vi "TEST - Delete Elements from 2D Array.vi"(8 "error in (no error)":errorcluster) -> (0 "error out":errorcluster, 2 "Pass?":bool=TRUE)   [LabVIEW 2009]
doc: "This VI template can be used for the functional testing of VIs; this implementation includes handling for the testing of polymorphic VIs, and the polymorphic elements should be removed if not needed.\n\nCoded by Douglas A. Femec, January 24, 2006.\n\nCopyright (c) 2005-2006 MKS Instruments, Inc.\nAll rights reserved."
uses:
  TEST - Delete Elements from 2D Array - Inputs.ctl
  Polymorphizer+ Data Type.ctl
  TEST - Delete Elements from 2D Array - Outputs.ctl
  source/library/Delete Elements from Array/Delete Elements from 2D Array (EXT).vi
  source/library/Delete Elements from Array/Delete Elements from 2D Array (I64).vi
  source/library/Delete Elements from Array/Delete Elements from 2D Array (U64).vi
  source/library/Delete Elements from Array/Delete Elements from 2D Array (DBL).vi
  source/library/Delete Elements from Array/Delete Elements from 2D Array (SGL).vi
  source/library/Delete Elements from Array/Delete Elements from 2D Array (I32).vi
  source/library/Delete Elements from Array/Delete Elements from 2D Array (I16).vi
  source/library/Delete Elements from Array/Delete Elements from 2D Array (I8).vi
  source/library/Delete Elements from Array/Delete Elements from 2D Array (LVObject).vi
  source/library/Delete Elements from Array/Delete Elements from 2D Array (U32).vi
  source/library/Delete Elements from Array/Delete Elements from 2D Array (U16).vi
  source/library/Delete Elements from Array/Delete Elements from 2D Array (U8).vi
  source/library/Delete Elements from Array/Delete Elements from 2D Array (CXT).vi
  source/library/Delete Elements from Array/Delete Elements from 2D Array (CDB).vi
  source/library/Delete Elements from Array/Delete Elements from 2D Array (CSG).vi
  source/library/Delete Elements from Array/Delete Elements from 2D Array (Boolean).vi
  source/library/Delete Elements from Array/Delete Elements from 2D Array (String).vi
  source/library/Delete Elements from Array/Delete Elements from 2D Array (Path).vi
  source/library/Delete Elements from Array/Delete Elements from 2D Array (Variant).vi
  TestClass/TestClass.lvclass
panel:
  out "Generated Outputs":T1[][](array[typedef])=[[{"Description"="expect empty array", "array w/ subset deleted"=[], "deleted elements"=[]}, {"Description"="expect empty array", "array w/ subset deleted"=[], "deleted elements"=[]}, {"Description"="expect empty array", "array w/ subset deleted"=[], "deleted elements"=[]}, {"Description"="expect empty array", "array w/ subset deleted"=[], "deleted elements"=[]}, {"Description"="expect empty array", "array w/ subset deleted"=[], "deleted elements"=[]}, {"Description"="expect empty array", "array w/ subset deleted"=[], "deleted elements"=[]}, {"Description"="expect empty array", "array w/ subset deleted"=[], "deleted elements"=[]}, {"Description"="expect empty array", "array w/ subset deleted"=[], "deleted elements"=[]}, {"Description"="expect empty array", "array w/ subset deleted"=[], "deleted elements"=[]}, {"Description"="expect empty array", "array w/ subset deleted"=[], "deleted elements"=[]}, {"Description"="expect empty array", "array w/ subset deleted"=[], "deleted elements"=[]}, {"Description"="expect empty array", "array w/ subset deleted"=[], "deleted elements"=[]}, {"Description"="expect empty array", "array w/ subset deleted"=[], "deleted elements"=[]}, {"Description"="expect empty array", "array w/ subset deleted"=[], "deleted elements"=[]}, {"Description"="expect empty array", "array w/ subset deleted"=[], "deleted elements"=[]}, {"Description"="expect empty array", "array w/ subset deleted"=[], "deleted elements"=[]}], [{"Description"="Some rows deleted", "array w/ subset deleted"=[[3.0, 4.0], [7.0, 8.0]], "deleted elements"=[[5.0, 6.0], [1.0, 2.0]]}, {"Description"="Some rows deleted", "array w/ subset deleted"=[[3.0, 4.0], [7.0, 8.0]], "deleted elements"=[[5.0, 6.0], [1.0, 2.0]]}, {"Description"="Some rows deleted", "array w/ subset deleted"=[[3.0, 4.0], [7.0, 8.0]], "deleted elements"=[[5.0, 6.0], [1.0, 2.0]]}, {"Description"="Some rows deleted", "array w/ subset deleted"=[[3.0, 4.0], [7.0, 8.0]], "deleted elements"=[[5.0, 6.0], [1.0, 2.0]]}, {"Description"="Some rows deleted", "array w/ subset deleted"=[[3.0, 4.0], [7.0, 8.0]], "deleted elements"=[[5.0, 6.0], [1.0, 2.0]]}, {"Description"="Some rows deleted", "array w/ subset deleted"=[[3.0, 4.0], [7.0, 8.0]], "deleted elements"=[[5.0, 6.0], [1.0, 2.0]]}, {"Description"="Some rows deleted", "array w/ subset deleted"=[[3.0, 4.0], [7.0, 8.0]], "deleted elements"=[[5.0, 6.0], [1.0, 2.0]]}, {"Description"="Some rows deleted", "array w/ subset deleted"=[[3.0, 4.0], [7.0, 8.0]], "deleted elements"=[[5.0, 6.0], [1.0, 2.0]]}, {"Description"="Some rows deleted", "array w/ subset deleted"=[[3.0, 4.0], [7.0, 8.0]], "deleted elements"=[[5.0, 6.0], [1.0, 2.0]]}, {"Description"="Some rows deleted", "array w/ subset deleted"=[[3.0, 4.0], [7.0, 8.0]], "deleted elements"=[[5.0, 6.0], [1.0, 2.0]]}, {"Description"="Some rows deleted", "array w/ subset deleted"=[[3.0, 4.0], [7.0, 8.0]], "deleted elements"=[[5.0, 6.0], [1.0, 2.0]]}, {"Description"="Some rows deleted", "array w/ subset deleted"=[[3.0, 4.0], [7.0, 8.0]], "deleted elements"=[[5.0, 6.0], [1.0, 2.0]]}, {"Description"="Some rows deleted", "array w/ subset deleted"=[[3.0, 4.0], [7.0, 8.0]], "deleted elements"=[[5.0, 6.0], [1.0, 2.0]]}, {"Description"="Some rows deleted", "array w/ subset deleted"=[[3.0, 4.0], [7.0, 8.0]], "deleted elements"=[[5.0, 6.0], [1.0, 2.0]]}, {"Description"="Some rows deleted", "array w/ subset deleted"=[[3.0, 4.0], [7.0, 8.0]], "deleted elements"=[[5.0, 6.0], [1.0, 2.0]]}, {"Description"="", "array w/ subset deleted"=[], "deleted elements"=[]}], [{"Description"="", "array w/ subset deleted"=[], "deleted elements"=[]}, {"Description"="", "array w/ subset deleted"=[], "deleted elements"=[]}, {"Description"="", "array w/ subset deleted"=[], "deleted elements"=[]}, {"Description"="", "array w/ subset deleted"=[], "deleted elements"=[]}, {"Description"="", "array w/ subset deleted"=[], "deleted elements"=[]}, {"Description"="", "array w/ subset deleted"=[], "deleted elements"=[]}, {"Description"="", "array w/ subset deleted"=[], "deleted elements"=[]}, {"Description"="", "array w/ subset deleted"=[], "deleted elements"=[]}, {"Description"="", "array w/ subset deleted"=[], "deleted elements"=[]}, {"Description"="", "array w/ subset deleted"=[], "deleted elements"=[]}, {"Description"="", "array w/ subset deleted"=[], "deleted elements"=[]}, {"Description"="", "array w/ subset deleted"=[], "deleted elements"=[]}, {"Description"="", "array w/ subset deleted"=[], "deleted elements"=[]}, {"Description"="", "array w/ subset deleted"=[], "deleted elements"=[]}, {"Description"="", "array w/ subset deleted"=[], "deleted elements"=[]}, {"Description"="", "array w/ subset deleted"=[], "deleted elements"=[]}], [{"Description"="", "array w/ subset deleted"=[], "deleted elements"=[]}, {"Description"="", "array w/ subset deleted"=[], "deleted elements"=[]}, {"Description"="", "array w/ subset deleted"=[], "deleted elements"=[]}, {"Description"="", "array w/ subset deleted"=[], "deleted elements"=[]}, {"Description"="", "array w/ subset deleted"=[], "deleted elements"=[]}, {"Description"="", "array w/ subset deleted"=[], "deleted elements"=[]}, {"Description"="", "array w/ subset deleted"=[], "deleted elements"=[]}, {"Description"="", "array w/ subset deleted"=[], "deleted elements"=[]}, {"Description"="", "array w/ subset deleted"=[], "deleted elements"=[]}, {"Description"="", "array w/ subset deleted"=[], "deleted elements"=[]}, {"Description"="", "array w/ subset deleted"=[], "deleted elements"=[]}, {"Description"="", "array w/ subset deleted"=[], "deleted elements"=[]}, {"Description"="", "array w/ subset deleted"=[], "deleted elements"=[]}, {"Description"="", "array w/ subset deleted"=[], "deleted elements"=[]}, {"Description"="", "array w/ subset deleted"=[], "deleted elements"=[]}, {"Description"="", "array w/ subset deleted"=[], "deleted elements"=[]}]] {"deleted elements" format="%.2f"; "array w/ subset deleted" format="%.2f"}
  in  "Expected Outputs":T1[](array[typedef])=[{"Description"="expect empty array", "array w/ subset deleted"=[], "deleted elements"=[]}, {"Description"="Some rows deleted", "array w/ subset deleted"=[[3.0, 4.0], [7.0, 8.0]], "deleted elements"=[[5.0, 6.0], [1.0, 2.0]]}, {"Description"="", "array w/ subset deleted"=[], "deleted elements"=[]}, {"Description"="", "array w/ subset deleted"=[], "deleted elements"=[]}] {"deleted elements" format="%.2f"; "array w/ subset deleted" format="%.2f"}
  in  "Inputs":T2[](array[typedef])=[{"Description"="Empty array", "Data Types to Test"=[enum."EXT", enum."DBL", enum."SGL", enum."I32", enum."I16", enum."I8", enum."U32", enum."U16", enum."U8", enum."CXT", enum."CDB", enum."CSG", enum."Boolean", enum."String", enum."Path", enum."Variant", enum."I64", enum."U64", enum."LabVIEW Object"], "Array"=[], "Indices"=[], "delete (rows or columns)"=enum."rows"}, {"Description"="Delete some rows", "Data Types to Test"=[enum."EXT", enum."DBL", enum."SGL", enum."I32", enum."I16", enum."I8", enum."U32", enum."U16", enum."U8", enum."CXT", enum."CDB", enum."CSG", enum."String", enum."Path", enum."Variant", enum."I64", enum."U64", enum."LabVIEW Object"], "Array"=[[1.0, 2.0], [3.0, 4.0], [5.0, 6.0], [7.0, 8.0]], "Indices"=[2, 0], "delete (rows or columns)"=enum."rows"}, {"Description"="", "Data Types to Test"=[enum."EXT", enum."DBL", enum."SGL", enum."I32", enum."I16", enum."I8", enum."U32", enum."U16", enum."U8", enum."CXT", enum."CDB", enum."CSG", enum."Boolean", enum."String", enum."Path", enum."Variant", enum."I64", enum."U64", enum."LabVIEW Object"], "Array"=[], "Indices"=[], "delete (rows or columns)"=enum."rows"}, {"Description"="", "Data Types to Test"=[enum."EXT", enum."DBL", enum."SGL", enum."I32", enum."I16", enum."I8", enum."U32", enum."U16", enum."U8", enum."CXT", enum."CDB", enum."CSG", enum."Boolean", enum."String", enum."Path", enum."Variant", enum."I64", enum."U64", enum."LabVIEW Object"], "Array"=[], "Indices"=[], "delete (rows or columns)"=enum."rows"}] {"Array" format="%.2f"}
  # "Copyright (c) 2005-2006 MKS Instruments, Inc.\nAll rights reserved."
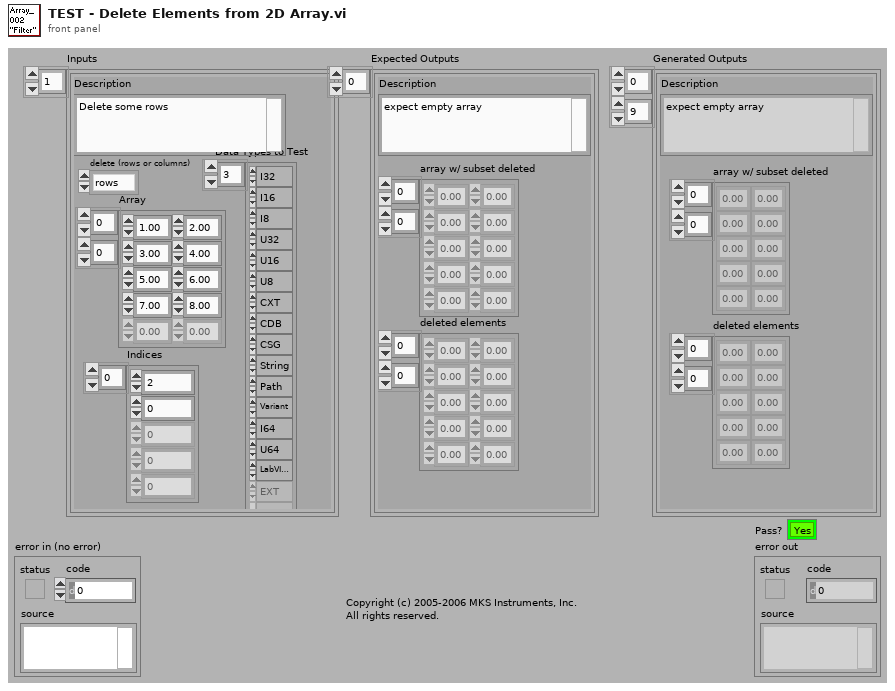
[diagram p1: front panel]
types:
  T1 = typedef "TEST - Delete Elements from 2D Array - Outputs.ctl" = cluster{"Description":string, "array w/ subset deleted":sgl[][], "deleted elements":sgl[][]}
  T2 = typedef "TEST - Delete Elements from 2D Array - Inputs.ctl" = cluster{"Description":string, "Data Types to Test":T3[], "Array":sgl[][], "Indices":i32[], "delete (rows or columns)":enum16{"rows", "columns"}}
  T3 = typedef "Polymorphizer+ Data Type.ctl" = enum16{"EXT", "DBL", "SGL", "I32", "I16", "I8", "U32", "U16", "U8", "CXT", "CDB", "CSG", "Boolean", "String", "Path", "Variant", "CTL-REF", "GEN-REF", "GObj-REF", "VI-REF", "ENUM", "ERR", "FILE-REF", "MENU-REF", "MENU-RING", "PICT-RING", "TXT&PICT-RING", "TXT-RING", "I64", "U64", "LabVIEW Object"}
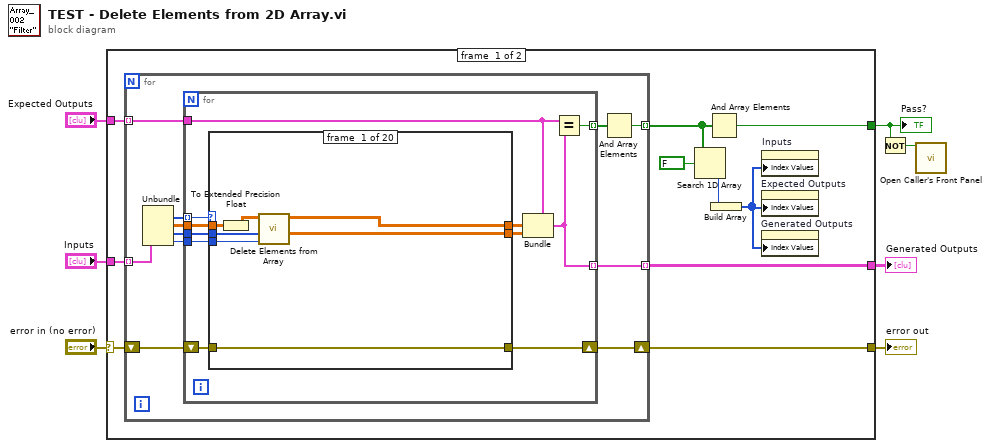
[diagram p0: block diagram]
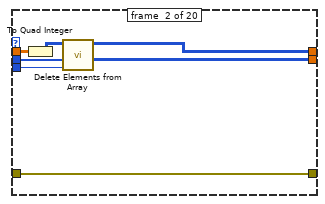
[diagram p2: hidden frame]
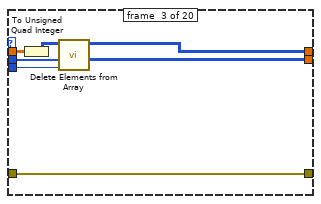
[diagram p3: hidden frame]
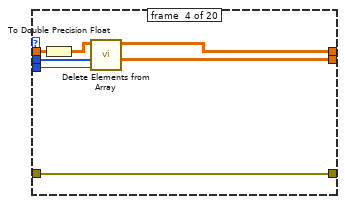
[diagram p4: hidden frame]
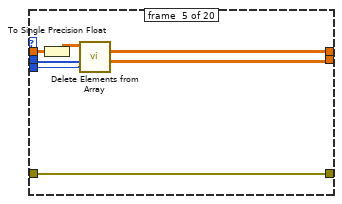
[diagram p5: hidden frame]
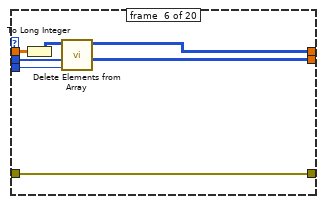
[diagram p6: hidden frame]
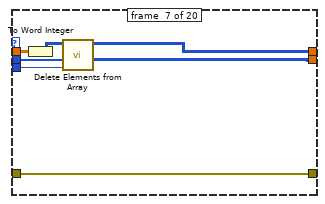
[diagram p7: hidden frame]
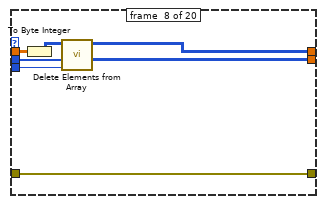
[diagram p8: hidden frame]
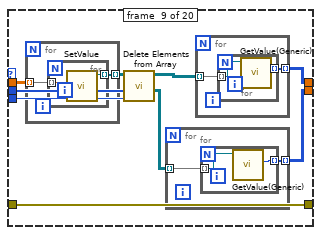
[diagram p9: hidden frame]
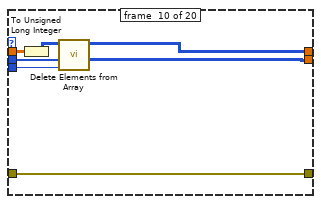
[diagram p10: hidden frame]
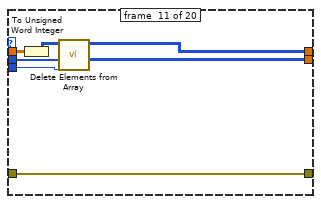
[diagram p11: hidden frame]
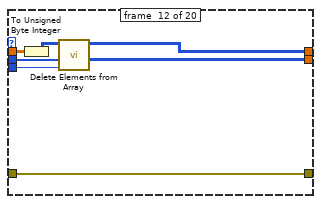
[diagram p12: hidden frame]
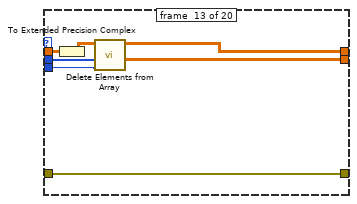
[diagram p13: hidden frame]
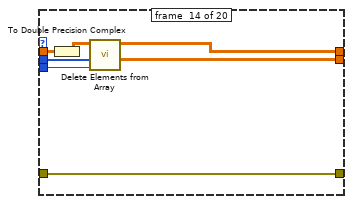
[diagram p14: hidden frame]
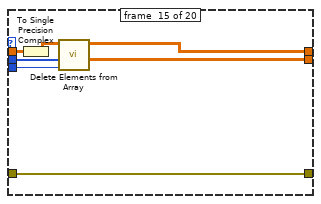
[diagram p15: hidden frame]
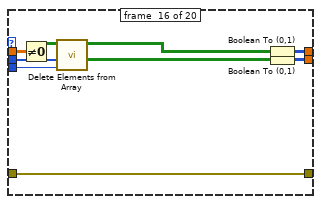
[diagram p16: hidden frame]
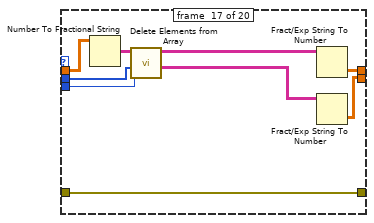
[diagram p17: hidden frame]
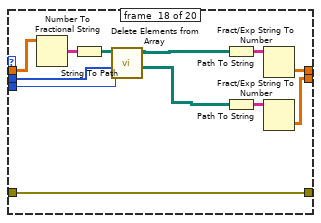
[diagram p18: hidden frame]
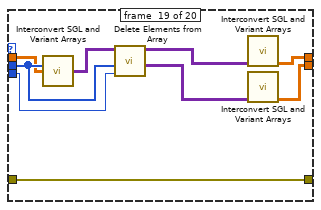
[diagram p19: hidden frame]
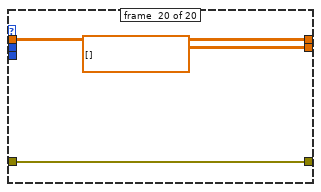
[diagram p20: hidden frame]
diagram:
  n1 = case shown="No Error" "error in (no error)" {
    selector: "error in (no error)" -> [w16 w201]
    tunnel: [w17 w201] -> w6
    tunnel: "Expected Outputs" -> [w14 _]
    tunnel: "Inputs" -> [w15 _]
    tunnel: [w13 _] -> w3
    tunnel: [w12 _] -> w2
    frame #0 {
      n2 = for {
        shift-right: [w23] -> w17
        shift-left: w16 -> [w24]
        tunnel: w15 -> [w25] mode=indexing
        tunnel: w14 -> [w28] mode=indexing
        tunnel: [w27] -> w13 mode=indexing
        tunnel: [w22] -> w11 mode=indexing
        n3 = Unbundle(w25) -> ("Data Types to Test"=w21:T3[], "Array"=w19:sgl[][], "Indices"=w20:i32[], "delete (rows or columns)"=w18:enum16{"rows", "columns"})  [unwired: 1 out]
        n4 = for {
          tunnel: w28 -> [w39]
          tunnel: [w37] -> w27 mode=indexing
          tunnel: [w38] -> w26 mode=indexing
          shift-right: [w32] -> w23
          shift-left: w24 -> [w33]
          tunnel: w21 -> [w34] mode=indexing
          tunnel: w19 -> [w36]
          tunnel: w20 -> [w35]
          tunnel: w18 -> [w29]
          n5 = case shown="\"LabVIEW Object\"" w34 {
            tunnel: w36 -> [w46 w53 w60 w67 w74 w81 w88 w95 w101 w123 w130 w137 w144 w151 w158 w167 w176 w187 w195 w199]
            tunnel: [w42 w49 w56 w63 w70 w77 w83 w90 w98 w118 w125 w132 w139 w146 w153 w166 w175 w186 w190 w199] -> w31
            tunnel: w35 -> [w43 w50 w57 w65 w71 w79 w86 w93 w103 w121 w128 w135 w142 w149 w156 w163 w173 w183 w196 _]
            tunnel: w33 -> [w45 w52 w59 w66 w73 w80 w87 w94 w104 w122 w129 w136 w143 w150 w157 w165 w174 w184 w197 w200]
            tunnel: [w45 w52 w59 w66 w73 w80 w87 w94 w104 w122 w129 w136 w143 w150 w157 w165 w174 w184 w197 w200] -> w32
            tunnel: [w41 w48 w55 w62 w69 w76 w84 w91 w96 w119 w126 w133 w140 w147 w154 w161 w169 w178 w191 cxt[][] []] -> w30
            tunnel: w29 -> [w40 w47 w54 w61 w68 w75 w82 w89 w102 w117 w124 w131 w138 w145 w152 w159 w168 w177 w189 _]
            frame #0 {
              n6 = To Extended Precision Float(1:w46) -> (0:w44:ext[][])
              n7 = call-poly "Delete Elements from Array.vi"("delete (rows or columns)"=w40, "indices"=w43, "array"=w44) -> ("deleted elements"=w41:ext[][], "array w/ subset deleted"=w42:ext[][])  [unwired: 7 in]
            }
            frame #1 {
              n8 = To Quad Integer(1:w53) -> (0:w51:i64[][])
              n9 = call-poly "Delete Elements from Array.vi"("delete (rows or columns)"=w47, "indices"=w50, "array"=w51) -> ("deleted elements"=w48:i64[][], "array w/ subset deleted"=w49:i64[][])  [unwired: 7 in]
            }
            frame #2 {
              n10 = To Unsigned Quad Integer(1:w60) -> (0:w58:u64[][])
              n11 = call-poly "Delete Elements from Array.vi"("delete (rows or columns)"=w54, "indices"=w57, "array"=w58) -> ("deleted elements"=w55:u64[][], "array w/ subset deleted"=w56:u64[][])  [unwired: 7 in]
            }
            frame #3 {
              n12 = To Double Precision Float(number=w67) -> (double precision float=w64:dbl[][])
              n13 = call-poly "Delete Elements from Array.vi"("delete (rows or columns)"=w61, "indices"=w65, "array"=w64) -> ("deleted elements"=w62:dbl[][], "array w/ subset deleted"=w63:dbl[][])  [unwired: 7 in]
            }
            frame #4 {
              n14 = To Single Precision Float(number=w74) -> (single precision float=w72:sgl[][])
              n15 = call-poly "Delete Elements from Array.vi"("delete (rows or columns)"=w68, "indices"=w71, "array"=w72) -> ("deleted elements"=w69:sgl[][], "array w/ subset deleted"=w70:sgl[][])  [unwired: 7 in]
            }
            frame #5 {
              n16 = To Long Integer(number=w81) -> (32bit integer=w78:i32[][])
              n17 = call-poly "Delete Elements from Array.vi"("delete (rows or columns)"=w75, "indices"=w79, "array"=w78) -> ("deleted elements"=w76:i32[][], "array w/ subset deleted"=w77:i32[][])  [unwired: 7 in]
            }
            frame #6 {
              n18 = To Word Integer(number=w88) -> (16bit integer=w85:i16[][])
              n19 = call-poly "Delete Elements from Array.vi"("delete (rows or columns)"=w82, "indices"=w86, "array"=w85) -> ("deleted elements"=w84:i16[][], "array w/ subset deleted"=w83:i16[][])  [unwired: 7 in]
            }
            frame #7 {
              n20 = To Byte Integer(number=w95) -> (8bit integer=w92:i8[][])
              n21 = call-poly "Delete Elements from Array.vi"("delete (rows or columns)"=w89, "indices"=w93, "array"=w92) -> ("deleted elements"=w91:i8[][], "array w/ subset deleted"=w90:i8[][])  [unwired: 7 in]
            }
            frame #8 {
              n22 = for {
                tunnel: w101 -> [w114] mode=indexing
                tunnel: [w113] -> w100 mode=indexing
                n23 = for {
                  tunnel: w114 -> [w116] mode=indexing
                  tunnel: [w115] -> w113 mode=indexing
                  n24 = call "SetValue.vi"("Value"=w116) -> ("TestClass out"=w115:refnum<class "TestClass.lvclass">)  [unwired: 9 in, 1 out]
                }
              }
              n25 = call-poly "Delete Elements from Array.vi"("delete (rows or columns)"=w102, "indices"=w103, "array"=w100) -> ("deleted elements"=w97:refnum<class>[][], "array w/ subset deleted"=w99:refnum<class>[][])  [unwired: 7 in]
              n26 = for {
                tunnel: w97 -> [w106] mode=indexing
                tunnel: [w105] -> w96 mode=indexing
                n27 = for {
                  tunnel: w106 -> [w107] mode=indexing
                  tunnel: [w108] -> w105 mode=indexing
                  n28 = call "GetValue(Generic).vi"("TestClass in"=w107) -> ("Value"=w108:i32)  [unwired: 8 in, 2 out]
                }
              }
              n29 = for {
                tunnel: w99 -> [w110] mode=indexing
                tunnel: [w109] -> w98 mode=indexing
                n30 = for {
                  tunnel: w110 -> [w111] mode=indexing
                  tunnel: [w112] -> w109 mode=indexing
                  n31 = call "GetValue(Generic).vi"("TestClass in"=w111) -> ("Value"=w112:i32)  [unwired: 8 in, 2 out]
                }
              }
            }
            frame #9 {
              n32 = To Unsigned Long Integer(number=w123) -> (unsigned 32bit integer=w120:u32[][])
              n33 = call-poly "Delete Elements from Array.vi"("delete (rows or columns)"=w117, "indices"=w121, "array"=w120) -> ("deleted elements"=w119:u32[][], "array w/ subset deleted"=w118:u32[][])  [unwired: 7 in]
            }
            frame #10 {
              n34 = To Unsigned Word Integer(number=w130) -> (unsigned 16bit integer=w127:u16[][])
              n35 = call-poly "Delete Elements from Array.vi"("delete (rows or columns)"=w124, "indices"=w128, "array"=w127) -> ("deleted elements"=w126:u16[][], "array w/ subset deleted"=w125:u16[][])  [unwired: 7 in]
            }
            frame #11 {
              n36 = To Unsigned Byte Integer(number=w137) -> (unsigned 8bit integer=w134:u8[][])
              n37 = call-poly "Delete Elements from Array.vi"("delete (rows or columns)"=w131, "indices"=w135, "array"=w134) -> ("deleted elements"=w133:u8[][], "array w/ subset deleted"=w132:u8[][])  [unwired: 7 in]
            }
            frame #12 {
              n38 = To Extended Precision Complex(1:w144) -> (0:w141:cxt[][])
              n39 = call-poly "Delete Elements from Array.vi"("delete (rows or columns)"=w138, "indices"=w142, "array"=w141) -> ("deleted elements"=w140:cxt[][], "array w/ subset deleted"=w139:cxt[][])  [unwired: 7 in]
            }
            frame #13 {
              n40 = To Double Precision Complex(1:w151) -> (0:w148:cdb[][])
              n41 = call-poly "Delete Elements from Array.vi"("delete (rows or columns)"=w145, "indices"=w149, "array"=w148) -> ("deleted elements"=w147:cdb[][], "array w/ subset deleted"=w146:cdb[][])  [unwired: 7 in]
            }
            frame #14 {
              n42 = To Single Precision Complex(1:w158) -> (0:w155:csg[][])
              n43 = call-poly "Delete Elements from Array.vi"("delete (rows or columns)"=w152, "indices"=w156, "array"=w155) -> ("deleted elements"=w154:csg[][], "array w/ subset deleted"=w153:csg[][])  [unwired: 7 in]
            }
            frame #15 {
              n44 = Not Equal To 0?(x=w167) -> (x != 0?=w164:bool[][])
              n45 = call-poly "Delete Elements from Array.vi"("delete (rows or columns)"=w159, "indices"=w163, "array"=w164) -> ("deleted elements"=w160:bool[][], "array w/ subset deleted"=w162:bool[][])  [unwired: 7 in]
              n46 = Boolean To (0,1)(Boolean=w162) -> (0, 1=w166:i16[][])
              n47 = Boolean To (0,1)(Boolean=w160) -> (0, 1=w161:i16[][])
            }
            frame #16 {
              n48 = Number To Fractional String(number=w176) -> (F-format string=w172:string[][])  [unwired: 3 in]
              n49 = call-poly "Delete Elements from Array.vi"("delete (rows or columns)"=w168, "indices"=w173, "array"=w172) -> ("deleted elements"=w170:string[][], "array w/ subset deleted"=w171:string[][])  [unwired: 7 in]
              n50 = Fract/Exp String To Number(string=w171) -> (number=w175:dbl[][])  [unwired: 3 in, 1 out]
              n51 = Fract/Exp String To Number(string=w170) -> (number=w169:dbl[][])  [unwired: 3 in, 1 out]
            }
            frame #17 {
              n52 = Number To Fractional String(number=w187) -> (F-format string=w188:string[][])  [unwired: 3 in]
              n53 = String To Path(string=w188) -> (path=w182:path[][])
              n54 = call-poly "Delete Elements from Array.vi"("delete (rows or columns)"=w177, "indices"=w183, "array"=w182) -> ("deleted elements"=w179:path[][], "array w/ subset deleted"=w181:path[][])  [unwired: 7 in]
              n55 = Path To String(path=w181) -> (string=w185:string[][])
              n56 = Path To String(path=w179) -> (string=w180:string[][])
              n57 = Fract/Exp String To Number(string=w185) -> (number=w186:dbl[][])  [unwired: 3 in, 1 out]
              n58 = Fract/Exp String To Number(string=w180) -> (number=w178:dbl[][])  [unwired: 3 in, 1 out]
            }
            frame #18 {
              n59 = call "Interconvert SGL and Variant Arrays.vi"("SGL 1D Array 2 In"=w196, "SGL 2D Array In"=w195) -> ("Variant 2D Array Out"=w194:variant[][])  [unwired: 9 in, 4 out]
              n60 = call-poly "Delete Elements from Array.vi"("delete (rows or columns)"=w189, "indices"=w196, "array"=w194) -> ("deleted elements"=w193:variant[][], "array w/ subset deleted"=w192:variant[][])  [unwired: 7 in]
              n61 = call "Interconvert SGL and Variant Arrays.vi"("Variant 2D Array In"=w192) -> ("SGL 2D Array Out"=w190:sgl[][])  [unwired: 10 in, 4 out]
              n62 = call "Interconvert SGL and Variant Arrays.vi"("Variant 2D Array In"=w193) -> ("SGL 2D Array Out"=w191:sgl[][])  [unwired: 10 in, 4 out]
            }
            frame #19 {
            }
          }
          n63 = Bundle(cluster=w39, "array w/ subset deleted"=w31, "deleted elements"=w30) -> (w37:T1)  [unwired: 1 in]
          n64 = Equal?(x=w39, y=w37) -> (x = y?=w38:bool)
        }
        n65 = And Array Elements(Boolean array=w26) -> (logical AND=w22:bool)
      }
      n66 = Search 1D Array(1D array=w11, element=FALSE) -> (index of element=w9:i32)  [unwired: 1 in]
      n67 = And Array Elements(Boolean array=w11) -> (logical AND=w12:bool)
      n68 = Build Array(w9) -> (w8:i32[])
      n69 = property on="Inputs" class="Arr (strict)"("Index Values"=w8) -> ()  [unwired: 2 in, 2 out]
      n70 = property on="Expected Outputs" class="Arr (strict)"("Index Values"=w8) -> ()  [unwired: 2 in, 2 out]
      n71 = property on="Generated Outputs" class="Arr (strict)"("Index Values"=w8) -> ()  [unwired: 2 in, 2 out]
    }
    frame #1 {
    }
  }
  "error out" <- w6
  "Pass?" <- w2
  "Generated Outputs" <- w3
  n72 = Not(x=w2) -> (.not. x?=w1:bool)
  n73 = call "Open Caller's Front Panel.vi"("Open?"=w1) -> ()  [unwired: 14 in, 1 out]
